vi "xiC - Tree_ValChange.vi"(8 "error in (no error)":errorcluster, 11 "Attributes In":T1) -> (0 "error out":errorcluster, 3 "Attributes Out":T1)   [LabVIEW 2013]
uses:
  xiC - Attributes.ctl
  C:/Projects/Cameras3.x/xiLib/xiLIB_64bit/xiLIB/xiCamLib/API/x64/xiApi.NETX64.dll
  xiLIB_64bit/xiLIB/xiCamLib/API/x64/xiApi.NETX64.dll
  xiC - TreeDisplayType.ctl
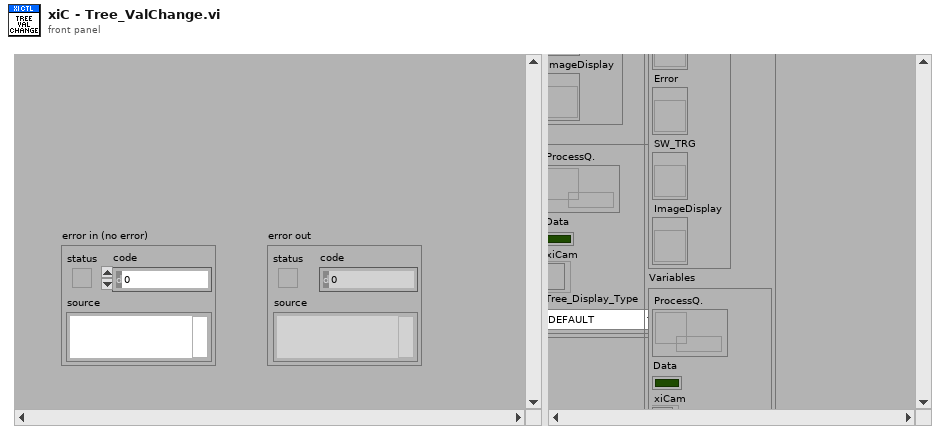
[diagram p1: front panel]
types:
  T1 = typedef "xiC - Attributes.ctl" = cluster{"Controls":cluster{"VI Ref.":refnum<vi>, "Tree":refnum<vi>, "Info":refnum<vi>, "PRMName":refnum<vi>, "xiControl":refnum<vi>, "Error":refnum<vi>, "SW_TRG":refnum<vi>, "ImageDisplay":refnum<vi>}, "Variables":cluster{"ProcessQ.":refnum<queue>, "Data":bool, "xiCam":refnum<k24>, "Tree_Display_Type":T2}}
  T2 = typedef "xiC - TreeDisplayType.ctl" = enum16{"DEFAULT", "HIDE_MAX_MIN"}
  T3 = typedef "PRM_v2.ctl" = enum16{"ACQ_BUFFER_SIZE", "ACQ_FRAME_BURST_COUNT", "ACQ_TIMING_MODE", "ACQ_TRANSPORT_BUFFER_SIZE", "AE_MAX_LIMIT", "AEAG", "AEAG_LEVEL", "API_VERSION", "AG_MAX_LIMIT", "APPLY_CMS", "AUTO_BANDWIDTH_CALCULATION", "AUTO_WB", "AVAILABLE_BANDWIDTH", "AVAILABLE_BANDWIDTH_MAX", "AVAILABLE_BANDWIDTH_MIN", "BPC", "BUFFER_POLICY", "BUFFERS_QUEUE_SIZE", "CC_MATRIX_00", "CC_MATRIX_01", "CC_MATRIX_02", "CC_MATRIX_03", "CC_MATRIX_10", "CC_MATRIX_11", "CC_MATRIX_12", "CC_MATRIX_13", "CC_MATRIX_20", "CC_MATRIX_21", "CC_MATRIX_22", "CC_MATRIX_23", "CC_MATRIX_30", "CC_MATRIX_31", "CC_MATRIX_32", "CC_MATRIX_33", "CHIP_TEMP", "CMS", "COLOR_FILTER_ARRAY", "COOLING", "DEBOUNCE_EN", "DEBOUNCE_POL", "DEBOUNCE_T0", "DEBOUNCE_T1", "DEBUG_LEVEL", "DEFAULT_CC_MATRIX", "DEVICE_INSTANCE_PATH", "DEVICE_MODEL_ID", "DEVICE_NAME", "DEVICE_SN", "DEVICE_TYPE", "DEVICE_USER_ID", "DOWNSAMPLING", "DOWNSAMPLING_MAX", "DOWNSAMPLING_MIN", "DOWNSAMPLING_TYPE", "DRV_VERSION", "EXP_PRIORITY", "EXPOSURE", "EXPOSURE_DIRECT_UPDATE", "EXPOSURE_MAX", "EXPOSURE_MIN", "FFS_FILE_NAME", "FPGA1_VERSION", "FRAMERATE", "FRAMERATE_MAX", "FRAMERATE_MIN", "FREE_FFS_SIZE", "GAIN", "GAIN_DIRECT_UPDATE", "GAIN_MAX", "GAIN_MIN", "GAMMAC", "GAMMAY", "GPI_LEVEL", "GPI_MODE", "GPI_SELECTOR", "GPI_SELECTOR_MAX", "GPI_SELECTOR_MIN", "GPO_MODE", "GPO_SELECTOR", "GPO_SELECTOR_MAX", "GPO_SELECTOR_MIN", "HDR", "HDR_T1", "HDR_T2", "HEIGHT", "HEIGHT_MAX", "HEIGHT_MIN", "HOUSE_TEMP", "IMAGE_DATA_FORMAT", "IMAGE_IS_COLOR", "INPUT_CMS_PROFILE", "IS_COOLED", "IS_DEVICE_EXIST", "KNEEPOINT1", "KNEEPOINT2", "LED_MODE", "LED_SELECTOR", "LED_SELECTOR_MAX", "LED_SELECTOR_MIN", "LIMIT_BANDWIDTH", "LIMIT_BANDWIDTH_MAX", "LIMIT_BANDWIDTH_MIN", "LUT_EN", "LUT_INDEX", "LUT_INDEX_MAX", "LUT_INDEX_MIN", "LUT_VALUE", "LUT_VALUE_MAX", "LUT_VALUE_MIN", "MANUAL_WB", "MCU1_VERSION", "MCU2_VERSION", "OFFSET_X", "OFFSET_X_MAX", "OFFSET_X_MIN", "OFFSET_Y", "OFFSET_Y_MAX", "OFFSET_Y_MIN", "OUTPUT_CMS_PROFILE", "OUTPUT_DATA_BIT_DEPTH", "OUTPUT_DATA_PACKING", "READ_FILE_FFS", "RECENT_FRAME", "SENSOR_DATA_BIT_DEPTH", "SENSOR_MODE", "SENSOR_TAPS", "SHARPNESS", "SHUTTER_TYPE", "TARGET_TEMP", "TRG_DELAY", "TRG_SELECTOR", "TRG_SOFTWARE", "TRG_SOURCE", "USED_FFS_SIZE", "WB_KB", "WB_KG", "WB_KR", "WIDTH", "WIDTH_MAX", "WIDTH_MIN", "WRITE_FILE_FFS", "ACQ_BUFFER_SIZE_UNIT", "ACQ_TRANSPORT_BUFFER_COMMIT", "AEAG_ROI_HEIGHT", "AEAG_ROI_OFFSET_X", "AEAG_ROU_OFFSET_Y", "AEAG_ROI_WIDTH", "API_CONTEXT_LIST", "BINNING_HORIZONTAL", "BINNING_PATTERN", "BINNING_SELECTOR", "BINNING_VERTICAL", "COLUMN_FPN_CORRECTION", "COUNTER_SELECTOR", "COUNTER_VALUE", "DECIMATION_HORIZONTAL", "DECIMATION_PATTERN", "DECIMATION_SELECTOR", "DECIMATION_VERTICAL", "DEVICE_ID", "DEVICE_LOCATION_PATH", "DEVICE_MANIFEST", "DEVICE_RESET", "DEVICE_SENS_SN", "EXPOSURE_BURST_COUNT", "FFS_ACCESS_KEY", "GAIN_SELECTOR", "HW_REVISION", "IMAGE_BLACK_LEVEL", "IMAGE_DATA_BIT_DEPTH", "IMAGE_DATA_FORMAT_RGB32_ALPHA", "IMAGE_PAYLOAD_SIZE", "LENS_APERTURE_VALUE", "LENS_FEATURE", "LENS_FEATURE_SELECTOR", "LENS_FOCAL_LENGTH", "LENS_FOCUS_DISTANCE", "LENS_FOCUS_MOVE", "LENS_FOCUS_MOVEMENT_VALUE", "LENS_MODE", "OUTPUT_DATA_PACKING_TYPE", "SENSOR_CLOCK_FREQ_HZ", "SENSOR_CLOCK_FREQ_INDEX", "SENSOR_FEATURE_SELECTOR", "SENSOR_FEATURE_VALUE", "SENSOR_OUTPUT_CHANNEL_COUNT", "TRANSPORT_PIXEL_FORMAT", "TS_RST_MODE", "TS_RST_SOURCE"}
  T4 = typedef "xiLIB - PRM_Attribute.ctl" = cluster{"Type":T5, "Method":T6, "Desc.":string, "PRM":T3}
  T5 = typedef "xiLIB - PRM_Type.ctl" = enum16{"Int32", "Float", "String", "DOWNSAMPLING_TYPE", "IMAGE_DATA_FORMAT", "BUFFER_POLICY", "TRG_SOURCE", "GPI", "GPO", "ACQ_TIMING_MODE", "BINNING_PATTERN", "BINNING_SELECTOR", "CMS_MODE", "COUNTER_SELECTOR", "DEBUG_LEVEL", "DECIMATION_PATTERN", "DECIMATION_SELECTOR", "GAIN_SELECTOR_TYPE", "LED_MODE", "LENS_FEATURE_SELECTOR", "LENS_MODE", "OUTPUT_DATA_PACKING_TYPE", "SENSOR_FEATURE_SELECTOR", "SHUTTER_TYPE", "TRG_SELECTOR", "TS_RST_MODE", "TS_RST_SOURCE"}
  T6 = typedef "xiLIB - PRM_Function.ctl" = enum16{"Get / Set", "Get", "Set"}
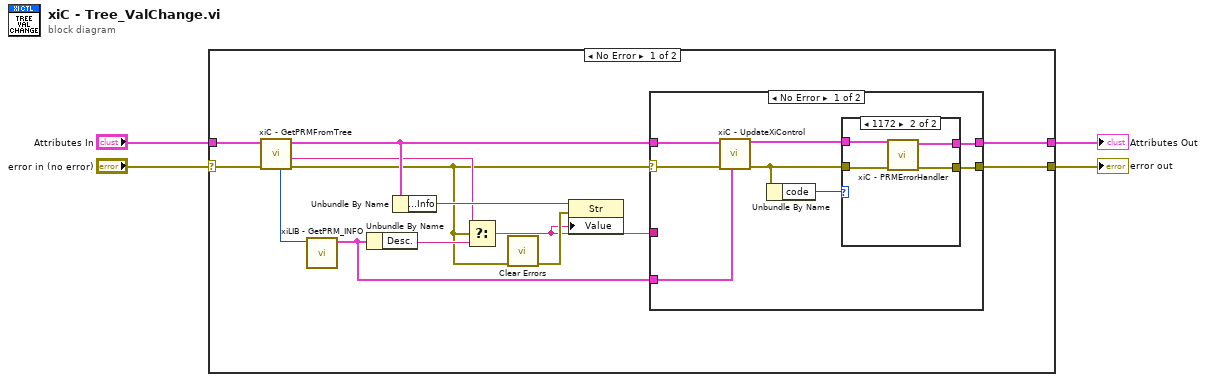
[diagram p0: block diagram]
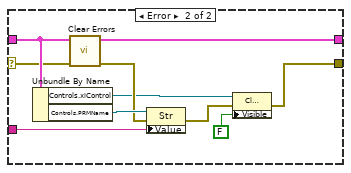
[diagram p3: hidden frame]
diagram:
  n1 = case shown="No Error" "error in (no error)" {
    selector: "error in (no error)" -> [w11 w42]
    tunnel: [w14 w42] -> w3
    tunnel: "Attributes In" -> [w13 w41]
    tunnel: [w15 w41] -> w1
    frame No Error {
      n2 = call "xiC - GetPRMFromTree.vi"("error in (no error)"=w11, "Attributes In"=w13) -> ("error out"=w6:errorcluster, "TreeValue"=w10:string, "Attributes Out"=w12:T1, "PRM"=w9:T3)  [unwired: 6 in]
      n3 = call "xiLIB - GetPRM_INFO.vi"("PRM"=w9) -> ("PRM_Attributes"=w7:T4)  [unwired: 10 in]
      n4 = Unbundle By Name(w7) -> ("Desc."=w8:string)
      n5 = Unbundle By Name(w12) -> ("Controls.Info"=w17:refnum<vi>)
      n6 = Select(t=w10, s=w6, f=w8) -> (s? t:f=w5:string)
      n7 = call <vilib>:"Clear Errors.vi"("error in (no error)"=w6) -> ("error out"=w16:errorcluster)  [unwired: 6 in]
      n8 = property class="Str"(reference=w17, error in=w16, "Value"=w5) -> ()  [unwired: 2 out]
      n9 = case shown="No Error" w6 {
        selector: w6 -> [w24 w39]
        tunnel: w12 -> [w25 w40]
        tunnel: [w19 w40] -> w15
        tunnel: [w18 w34] -> w14
        tunnel: w7 -> [w23 _]
        tunnel: w5 -> [_ w32]
        frame No Error {
          n10 = call "xiC - UpdateXiControl.vi"("PRM_Attributes"=w23, "error in (no error)"=w24, "Attributes In"=w25) -> ("error out"=w21:errorcluster, "Attributes Out"=w22:T1)  [unwired: 7 in]
          n11 = Unbundle By Name(w21) -> ("code"=w20:i32)
          n12 = case shown="1172" w20 {
            tunnel: w22 -> [w27 w31]
            tunnel: w21 -> [w26 w30]
            tunnel: [w27 w29] -> w19
            tunnel: [w26 w28] -> w18
            frame 0, Default {
            }
            frame 1172 {
              n13 = call "xiC - PRMErrorHandler.vi"("error in (no error)"=w30, "Attributes In"=w31) -> ("error out"=w28:errorcluster, "Attributes Out"=w29:T1)  [unwired: 8 in]
            }
          }
        }
        frame Error {
          n14 = Unbundle By Name(w40) -> ("Controls.xiControl"=w36:refnum<vi>, "Controls.PRMName"=w38:refnum<vi>)
          n15 = call <vilib>:"Clear Errors.vi"("error in (no error)"=w39) -> ("error out"=w37:errorcluster)  [unwired: 6 in]
          n16 = property class="Str"(reference=w38, error in=w37, "Value"=w32) -> (error out=w35:errorcluster)  [unwired: 1 out]
          n17 = property class="Clust (strict)"(reference=w36, error in=w35, "Visible"=FALSE) -> (error out=w34:errorcluster)  [unwired: 1 out]
        }
      }
    }
    frame Error {
    }
  }
  "error out" <- w3
  "Attributes Out" <- w1
